vi "Calibrate NART DUT_old.vi"(0 "RFSA Device":refnum<k15>="RFSA" caption="instrument handle", 1 "port":u16=3363, 2 "Host":string="10.234.39.192", 3 "CART TCP Connection In":refnum<k5>, 5 "Measurement Handle In":T4, 7 "Frequency and Tx Gain":cluster{"Frequency":u32, "TX Gain":u32}[](array[cluster]), 9 "Data Rates":string[](array[combo]), 11 "error in (no error)":errorcluster, 12 "External Attenuation, dB":T2 format="%.2f", 13 "Measurement Timeout, sec":T1=10.0 format="%.3f") -> (4 "RFSA Handle Out":T3="RFSA" caption="RFSA Handle", 6 "Measurement Handle Out":T4, 8 "CART TCP Connection Out":refnum<k5>, 15 "error out":errorcluster)   [LabVIEW 2011]
uses:
  <userlib>/niRF/niBasic/SA/Waveform/Includes/niBASIC - SA - Waveform - INC - STYP - Measurement Handle.ctl
  <userlib>/niRF/niBasic/SA/Waveform/Includes/niBASIC - SA - Waveform - INC - STYP - State Element.ctl
  <userlib>/niRF/niSystem/SA/Includes/niSYS - SA - INC - STYP - Measurement Interval.ctl
  <userlib>/niRF/niSystem/SA/Includes/niSYS - SA - INC - STYP - RBW Filter.ctl
  <userlib>/niRF/niSystem/SA/Includes/niSYS - SA - INC - STYP - External Attenuation.ctl
  <userlib>/niRF/niBasic/SA/Waveform/Includes/niBASIC - SA - Waveform - INC - STYP - Averaging.ctl
  <userlib>/niRF/niSystem/SA/Includes/niSYS - RFSA - INC - STYP - Handle.ctl
  <userlib>/niRF/niSystem/SA/Includes/niSYS - SA - INC - STYP - Timeout.ctl
  <userlib>/niRF/niSystem/SA/Includes/niSYS - SA - INC - STYP - Measurement Request.ctl
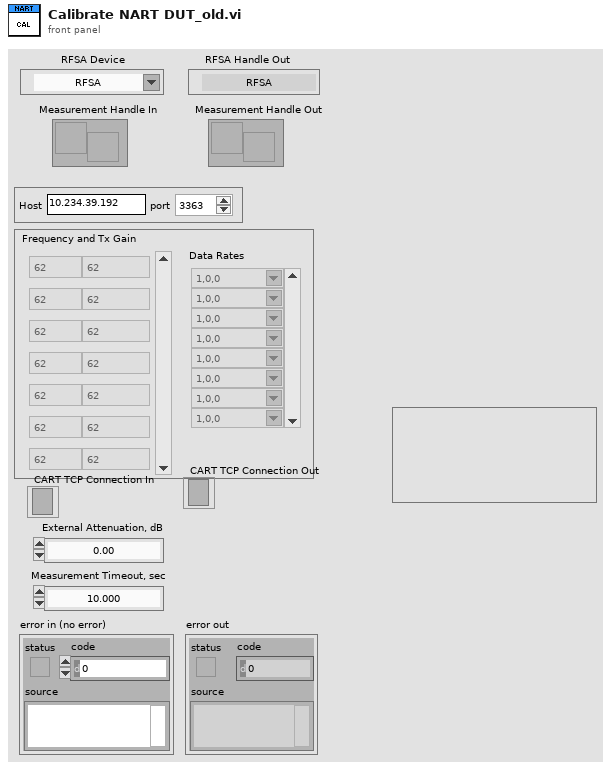
[diagram p1: front panel]
types:
  T1 = typedef "niSYS - SA - INC - STYP - Timeout.ctl" = dbl
  T2 = typedef "niSYS - SA - INC - STYP - External Attenuation.ctl" = dbl
  T3 = typedef "niSYS - RFSA - INC - STYP - Handle.ctl" = refnum<k15>
  T4 = typedef "niBASIC - SA - Waveform - INC - STYP - Measurement Handle.ctl" = refnum<notifier>
  T5 = typedef "niSYS - SA - INC - STYP - Measurement Interval.ctl" = dbl
  T6 = typedef "niSYS - SA - INC - STYP - Measurement Request.ctl" = enum16{"Measure", "Fetch", "Initiate"}
  T7 = cluster{"Frequency, MHz":u32, "TX Gain":u32, "Data Rate":string, "Packet Length":u32, "Packet Count":i32}
  T8 = typedef "niBASIC - SA - Waveform - INC - STYP - Measurement.ctl" = cluster{"Mean Power, dBm":dbl, "Peak to Average Ratio, dB":dbl, "Maximum Power, dBm":dbl, "Minimum Power, dBm":dbl}
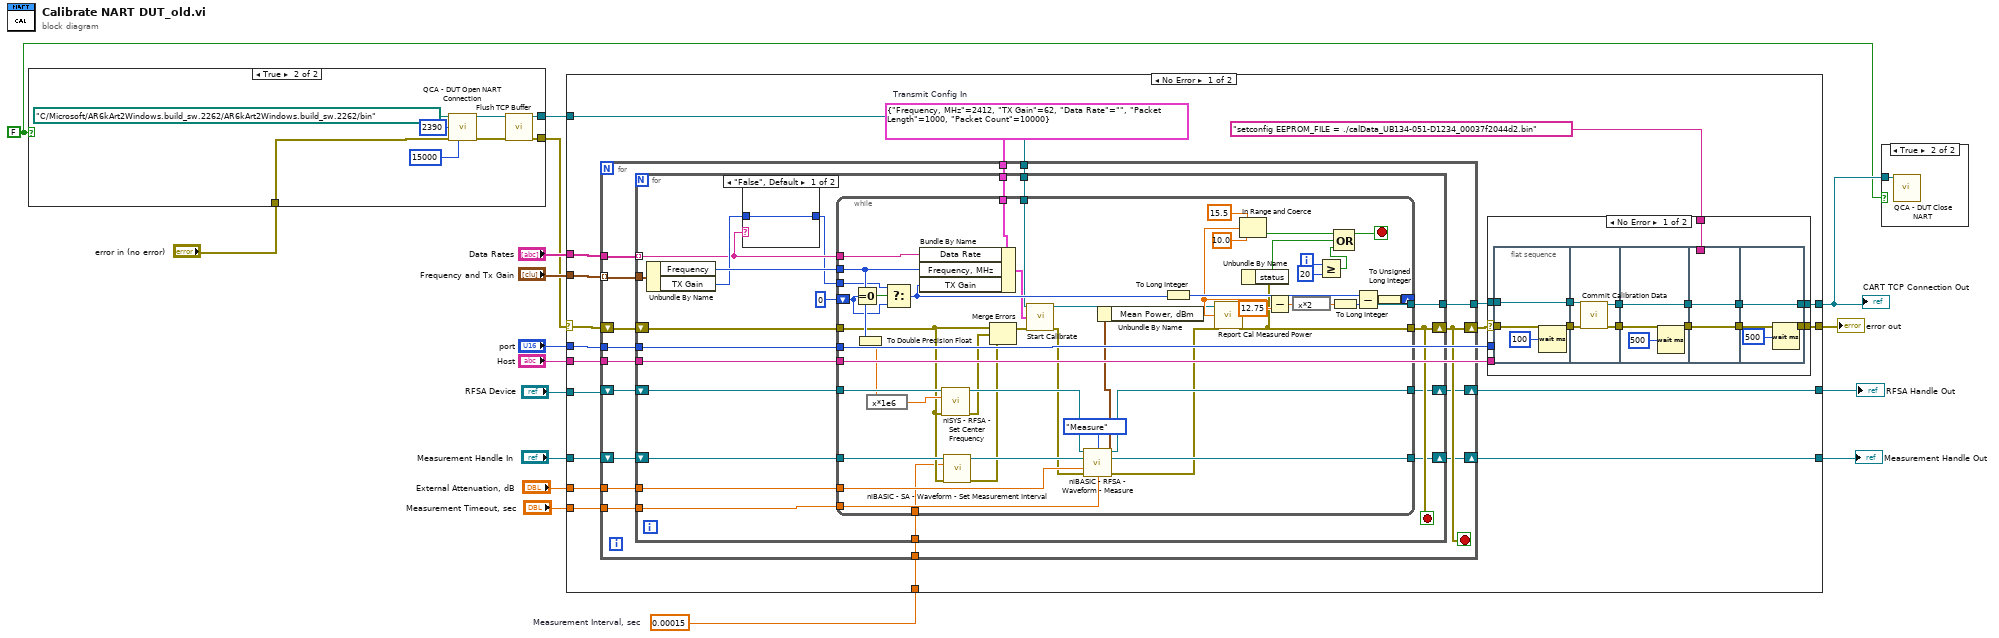
[diagram p0: block diagram]
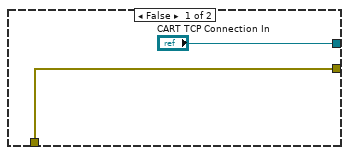
[diagram p3: hidden frame]
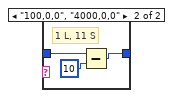
[diagram p5: hidden frame]
diagram:
  w1 = FALSE
  w6 = T5 0.00015  # Measurement Interval, sec
  n1 = case shown="True" w1 {
    tunnel: [w19 w22] -> w5
    tunnel: ["CART TCP Connection In" w21] -> w4
    tunnel: "error in (no error)" -> [w19 w20]
    frame False {
    }
    frame True {
      n2 = call "QCA - DUT Open NART Connection.vi"("NART Directory"=path "C:/Microsoft/AR6kArt2Windows.build_sw.2262/AR6kArt2Windows.build_sw.2262/bin", "port (2390)"=u32 2390, "error in (no error)"=w20, "Timeout (2500ms)"=15000) -> ("NART TCP Connection"=w24:refnum<k5>, "error out"=w23:errorcluster)  [unwired: 10 in]
      n3 = call "Flush TCP Buffer.vi"("CART TCP Connection In"=w24, "error in (no error)"=w23) -> ("CART TCP Connection Out"=w21:refnum<k5>, "error out"=w22:errorcluster)  [unwired: 12 in]
    }
  }
  n4 = case shown="No Error" w5 {
    selector: w5 -> [w42 w167]
    tunnel: [w43 w167] -> w15
    tunnel: "port" -> [w39 _]
    tunnel: "Host" -> [w40 _]
    tunnel: "Data Rates" -> [w45 _]
    tunnel: "Frequency and Tx Gain" -> [w44 _]
    tunnel: "Measurement Handle In" -> [w38 w165]
    tunnel: [w37 w165] -> w11
    tunnel: "RFSA Device" -> [w36 w166]
    tunnel: [w35 w166] -> w9
    tunnel: "External Attenuation, dB" -> [w34 _]
    tunnel: "Measurement Timeout, sec" -> [w33 _]
    tunnel: w6 -> [w32 _]
    tunnel: w4 -> [w31 w164]
    tunnel: [w29 w164] -> w3
    frame No Error {
      w46 = T7 {"Frequency, MHz"=2412, "TX Gain"=62, "Data Rate"="", "Packet Length"=1000, "Packet Count"=10000}  # Transmit Config In
      n5 = for {
        tunnel: w39 -> [w92]
        tunnel: w40 -> [w91]
        tunnel: w46 -> [w90]
        tunnel: w45 -> [w88]
        tunnel: w44 -> [w89] mode=indexing
        shift-right: [w87] -> w41
        shift-left: w42 -> [w86]
        shift-right: [w84] -> w37
        shift-left: w38 -> [w85]
        shift-right: [w82] -> w35
        shift-left: w36 -> [w83]
        tunnel: w34 -> [w81]
        tunnel: w33 -> [w80]
        tunnel: w32 -> [w79]
        tunnel: w31 -> [w78]
        tunnel: [w77] -> w30
        stop <- w87 stop-if-true
        n6 = for {
          tunnel: w92 -> [w110]
          tunnel: w91 -> [w108]
          tunnel: w90 -> [w112]
          tunnel: w89 -> [w111]
          tunnel: w88 -> [w96] mode=indexing
          shift-right: [w109] -> w87
          shift-left: w86 -> [w100]
          shift-right: [w106] -> w84
          shift-left: w85 -> [w107]
          shift-right: [w105] -> w82
          shift-left: w83 -> [w102]
          tunnel: w81 -> [w104]
          tunnel: w80 -> [w103]
          tunnel: w79 -> [w99]
          tunnel: w78 -> [w94]
          tunnel: [w93] -> w77
          stop <- w109 stop-if-true
          n7 = Unbundle By Name(w111) -> ("Frequency"=w101:u32, "TX Gain"=w97:u32)
          n8 = case shown="\"False\", Default" w96 {
            tunnel: w97 -> [w113 w116]
            tunnel: [w113 w114] -> w95
            frame "False", Default {
            }
            frame "100,0,0", "4000,0,0" {
              # "1 L, 11 S"
              n9 = Subtract(x=w116, y=u32 10) -> (x-y=w114:u32)
            }
          }
          n10 = while {
            tunnel: w112 -> [w163]
            tunnel: w96 -> [w162]
            tunnel: w110 -> [_]
            tunnel: [w124] -> w109
            tunnel: w108 -> [_]
            tunnel: w107 -> [w158]
            tunnel: [w157] -> w106
            tunnel: [w156] -> w105
            tunnel: w104 -> [w155]
            tunnel: w103 -> [w154]
            tunnel: w102 -> [w153]
            tunnel: w101 -> [w151]
            tunnel: w100 -> [w149]
            tunnel: w99 -> [w146]
            shift-right: [w132] -> _
            shift-left: u32 0 ("TX Gain") -> [w138]
            tunnel: w95 -> [w144]
            tunnel: w94 -> [w119]
            tunnel: [w117] -> w93
            i -> [w127]
            stop <- w131 stop-if-true
            n11 = Equal To 0?(x=w138) -> (x = 0?=w145:bool)
            n12 = To Double Precision Float(number=w151) -> (double precision float=w129:dbl)
            n13 = expression code="x*1e6"(w129) -> (w150:dbl)
            n14 = Select(t=w144, s=w145, f=w138) -> (s? t:f=w137:u32)
            n15 = Bundle By Name(cluster=w163, "Data Rate"=w162, "Frequency, MHz"=w151, "TX Gain"=w137) -> (w120:T7)
            n16 = call <userlib>:"niSYS - RFSA - Set Center Frequency.vi"("RFSA Handle In"=w153, "RFSA Center Frequency, Hz"=w150, "error in (no error)"=w149) -> ("RFSA Handle Out"=w152:T3, "error out"=w148:errorcluster)  [unwired: 11 out]
            n17 = call <userlib>:"niBASIC - SA - Waveform - Set Measurement Interval.vi"("Measurement Handle In"=w158, "Measurement Interval, sec"=w146, "error in (no error)"=w149) -> ("Measurement Handle Out"=w159:T4, "error out"=w147:errorcluster)  [unwired: 11 out]
            n18 = Merge Errors(w149, w148, w147) -> (w121:errorcluster)
            n19 = call "Start Calibrate.vi"("CART TCP Connection In"=w119, "Calibrate Config"=w120, "error in (no error)"=w121) -> ("CART TCP Connection Out"=w118:refnum<k5>, "error out"=w122:errorcluster)  [unwired: 9 in, 2 out]
            n20 = call <userlib>:"niBASIC - RFSA - Waveform - Measure.vi"("RFSA Handle In"=w152, "Measurement Request"=niSYS_-_SA_-_INC_-_STYP_-_Measurement_Request."Measure", "Measurement Handle In"=w159, "External Attenuation, dB"=w155, "error in (no error)"=w122, "Timeout, sec"=w154) -> ("RFSA Handle Out"=w156:T3, "Measurement Handle Out"=w157:T4, "Measurement"=w160:T8, "error out"=w125:errorcluster)  [unwired: 2 in, 4 out]
            n21 = Unbundle By Name(w160) -> ("Mean Power, dBm"=w123:dbl)
            n22 = To Long Integer(number=w137) -> (32bit integer=w134:i32)
            n23 = call "Report Cal Measured Power.vi"("CART TCP Connection In"=w118, "Measured Cal Power"=w123, "error in (no error)"=w125) -> ("CART TCP Connection Out"=w117:refnum<k5>, "error out"=w124:errorcluster)  [unwired: 9 in, 2 out]
            n24 = In Range and Coerce(upper limit=15.5, x=w123, lower limit=10.0) -> (In Range?=w141:bool)  [unwired: 1 out]
            n25 = Unbundle By Name(w124) -> ("status"=w130:bool)
            n26 = Subtract(x=w123, y=12.75) -> (x-y=w139:dbl)
            n27 = expression code="x*2"(w139) -> (w135:dbl)
            n28 = Greater Or Equal?(x=w127, y=20) -> (x >= y?=w128:bool)
            n29 = To Long Integer(number=w135) -> (32bit integer=w136:i32)
            n30 = Compound Arithmetic op=OR(w141, w130, w128) -> (w131:bool)
            n31 = Subtract(x=w134, y=w136) -> (x-y=w133:i32)
            n32 = To Unsigned Long Integer(number=w133) -> (unsigned 32bit integer=w132:u32)
          }
        }
      }
      n33 = case shown="No Error" w41 {
        selector: w41 -> [w59 w76]
        tunnel: [w58 w76] -> w43
        tunnel: w40 -> [_ _]
        tunnel: w39 -> [_ _]
        tunnel: w30 -> [w57 w75]
        tunnel: [w56 w75] -> w29
        tunnel: "setconfig EEPROM_FILE = ./calData_UB134-051-D1234_00037f2044d2.bin" ("Expected Message Start (\"\":any)") -> [w49 _]
        frame No Error {
          n34 = flat-sequence {
            tunnel: w57 -> [w61]
            tunnel: w59 -> [w62]
            tunnel: [w62] -> w55
            tunnel: [w61] -> w54
            tunnel: w55 -> [w66]
            tunnel: w54 -> [w64]
            tunnel: [w65] -> w53
            tunnel: [w63] -> w52
            tunnel: w53 -> [w69]
            tunnel: w52 -> [w68]
            tunnel: [w69] -> w51
            tunnel: [w68] -> w50
            tunnel: w51 -> [w71]
            tunnel: w50 -> [w70]
            tunnel: w49 -> [_]
            tunnel: [w71] -> w48
            tunnel: [w70] -> w47
            tunnel: [w73] -> w56
            tunnel: [w74] -> w58
            tunnel: w48 -> [w74]
            tunnel: w47 -> [w73]
            frame #0 {
              n35 = Wait (ms)(milliseconds to wait=u32 100) -> ()  [unwired: 1 out]
            }
            frame #1 {
              n36 = call "Commit Calibration Data.vi"("CART TCP Connection In"=w64, "error in (no error)"=w66) -> ("CART TCP Connection Out"=w63:refnum<k5>, "error out"=w65:errorcluster)  [unwired: 11 in, 1 out]
            }
            frame #2 {
              n37 = Wait (ms)(milliseconds to wait=u32 500) -> ()  [unwired: 1 out]
            }
            frame #3 {
            }
            frame #4 {
              n38 = Wait (ms)(milliseconds to wait=u32 500) -> ()  [unwired: 1 out]
            }
          }
        }
        frame Error {
        }
      }
    }
    frame Error {
    }
  }
  "error out" <- w15
  "Measurement Handle Out" <- w11
  "RFSA Handle Out" <- w9
  "CART TCP Connection Out" <- w3
  n39 = case shown="True" w1 {
    tunnel: w3 -> [_ w168]
    frame False {
    }
    frame True {
      n40 = call "QCA - DUT Close NART.vi"("CART TCP Connection"=w168) -> ()  [unwired: 14 in, 1 out]
    }
  }
